vi "main.vi"() -> ()   [LabVIEW 2021]
panel:
  in  "stop":bool
  out "Data":dbl(graph)
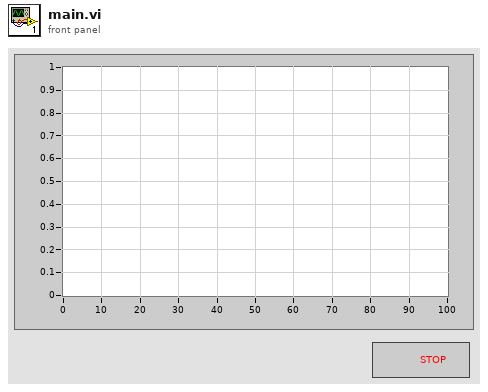
[diagram p1: front panel]
types:
  T1 = enum32{"invalid app kind", "Development System", "Run Time System", "Student Edition", "Embedded LabVIEW", "Evaluation", "Custom"}
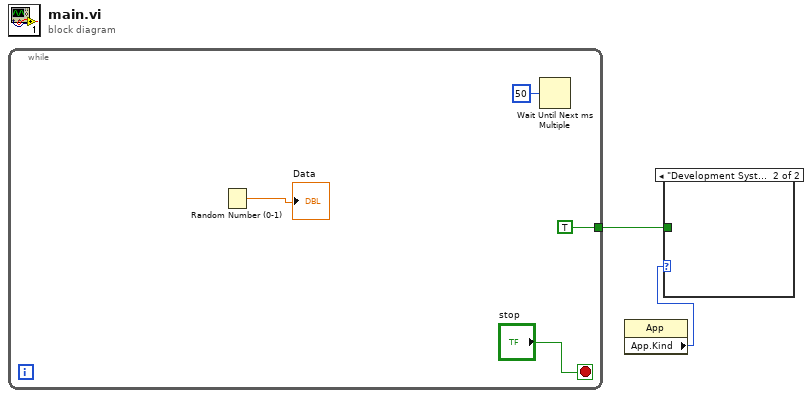
[diagram p0: block diagram]
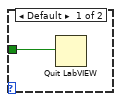
[diagram p2: hidden frame]
diagram:
  n1 = while {
    tunnel: [TRUE ("quit? (T)")] -> w2
    stop <- "stop" stop-if-true
    n2 = Random Number (0-1)() -> (number: 0 to 1=→"Data":dbl)
    n3 = Wait Until Next ms Multiple(millisecond multiple=u32 50) -> ()  [unwired: 1 out]
  }
  n4 = property class="App"() -> ("App.Kind"=w1:T1)  [unwired: 2 in, 2 out]
  n5 = case shown="\"Development System\"" w1 {
    tunnel: w2 -> [w7 _]
    frame Default {
      n6 = Quit LabVIEW(quit? (T)=w7) -> ()
    }
    frame "Development System" {
    }
  }
